vi "statsNsplit2ADC.vi"(4 "Start":i32=200, 5 "Tabin":i32[](array[numeric])=[0, 1, 2, 3, 4, 5, 6, 7, 8, 0, 1, 2, 3, 4, 5, 6, 7, 8], 6 "Nbins":i32=1, 7 "channel nb":u8=8 format="%x") -> (0 "Averages":dbl[][](array[numeric]), 1 "S.Dev.":dbl[][](array[numeric]), 2 "Minima":i32[][](array[numeric]), 3 "Maxima":i32[][](array[numeric]))   [LabVIEW 2014]
uses:
  <vilib>/Analysis/NI_AALBase.lvlib
panel:
  out "subarray":i32[](array[numeric])
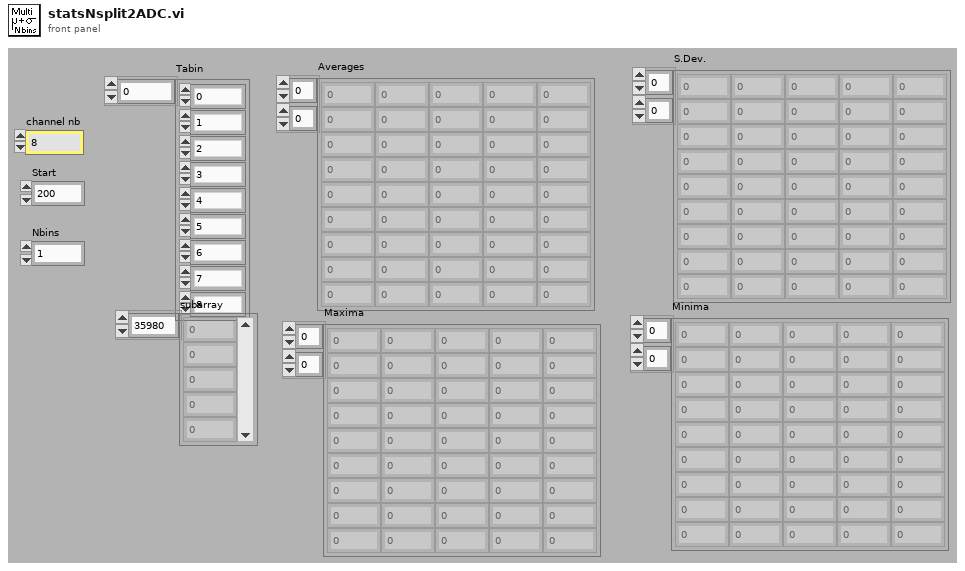
[diagram p1: front panel]
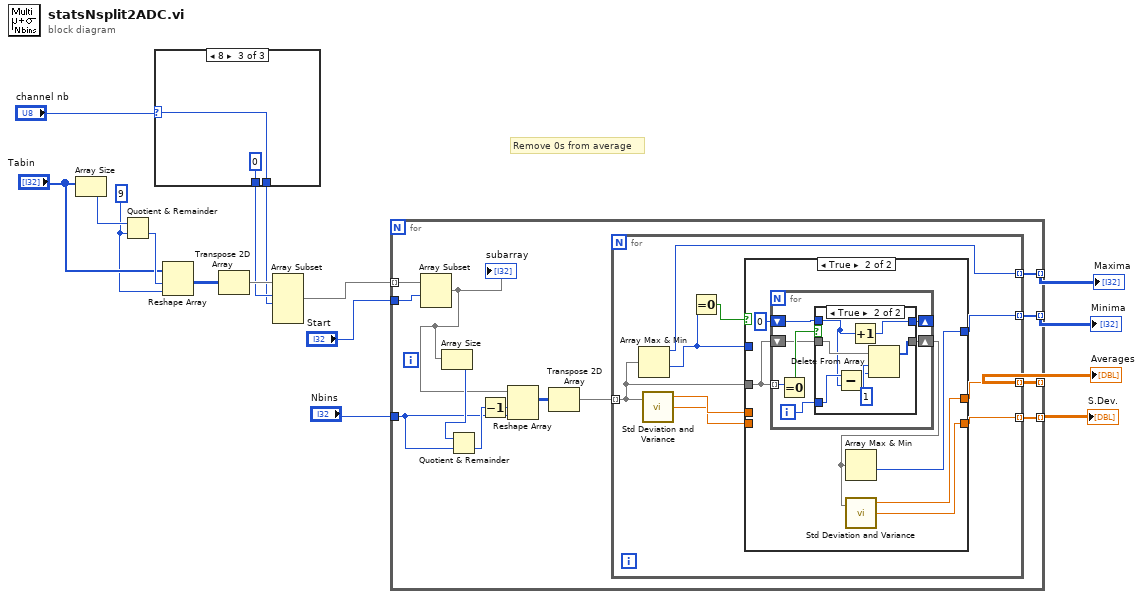
[diagram p0: block diagram]
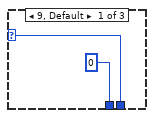
[diagram p2: hidden frame]
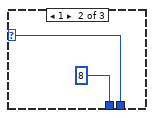
[diagram p3: hidden frame]
diagram:
  w7 = 9
  # "Remove 0s from average"
  n1 = Array Size(array="Tabin") -> (size(s)=w12:i32)
  n2 = Quotient & Remainder(x=w12, y=w7) -> (floor(x/y)=w11:i32)  [unwired: 1 out]
  n3 = case shown="8" "channel nb" {
    selector: "channel nb" -> [w17 w20 w22]
    tunnel: [w17 w20 w22] -> w3
    tunnel: [0 8 0] -> w4
    frame 9, Default {
    }
    frame 1 {
    }
    frame 8 {
    }
  }
  n4 = Reshape Array("Tabin", w11, w7) -> (w9:i32[][])
  n5 = Transpose 2D Array(2D array=w9) -> (transposed array=w8:i32[][])
  n6 = Array Subset(array=w8, index (row)=w4, length (row)=w3) -> (w6:i32[][])  [unwired: 2 in]
  n7 = for {
    tunnel: "Start" -> [w28]
    tunnel: "Nbins" -> [w30]
    tunnel: [w34] -> w14 mode=indexing
    tunnel: [w33] -> w13 mode=indexing
    tunnel: w6 -> [w27] mode=indexing
    tunnel: [w24] -> w2 mode=indexing
    tunnel: [w23] -> w1 mode=indexing
    n8 = Array Subset(array=w27, index=w28) -> (w26:i32[])  [unwired: 1 in]
    "subarray" <- w26
    n9 = Array Size(array=w26) -> (size(s)=w32:i32)
    n10 = Quotient & Remainder(x=w32, y=w30) -> (floor(x/y)=w31:i32)  [unwired: 1 out]
    n11 = Decrement(x=w31) -> (x-1=w25:i32)
    n12 = Reshape Array(w26, w25, w30) -> (w35:i32[][])
    n13 = Transpose 2D Array(2D array=w35) -> (transposed array=w29:i32[][])
    n14 = for {
      tunnel: w29 -> [w36] mode=indexing
      tunnel: [w39] -> w34 mode=indexing
      tunnel: [w37] -> w33 mode=indexing
      tunnel: [w43] -> w24 mode=indexing
      tunnel: [w41] -> w23 mode=indexing
      n15 = Array Max & Min(array=w36) -> (max value=w43:i32, min value=w42:i32)  [unwired: 2 out]
      n16 = call <vilib>:"Std Deviation and Variance.vi"("X"=w36) -> ("mean"=w40:dbl, "standard deviation"=w38:dbl)  [unwired: 1 in, 1 out]
      n17 = Equal To 0?(x=w42) -> (x = 0?=w44:bool)
      n18 = case shown="True" w44 {
        tunnel: w42 -> [w47 _]
        tunnel: [w47 w48] -> w41
        tunnel: w40 -> [w46 _]
        tunnel: [w46 w50] -> w39
        tunnel: w38 -> [w45 _]
        tunnel: [w45 w49] -> w37
        tunnel: w36 -> [_ w53]
        frame False {
        }
        frame True {
          n19 = for {
            tunnel: w53 -> [w60] mode=indexing
            shift-right: [w54] -> w51
            shift-left: w53 -> [w56]
            shift-right: [w57] -> _
            shift-left: 0 -> [w58]
            i -> [w55]
            n20 = Equal To 0?(x=w60) -> (x = 0?=w59:bool)
            n21 = case shown="True" w59 {
              tunnel: w58 -> [w62 w65]
              tunnel: [w62 w69] -> w57
              tunnel: w56 -> [w61 w68]
              tunnel: w55 -> [_ w66]
              tunnel: [w61 w63] -> w54
              frame False {
              }
              frame True {
                n22 = Subtract(x=w66, y=w65) -> (x-y=w64:i32)
                n23 = Increment(x=w65) -> (x+1=w69:i32)
                n24 = Delete From Array(array=w68, length=1, index=w64) -> (array with subset deleted=w63:i32[])  [unwired: 1 out]
              }
            }
          }
          n25 = Array Max & Min(array=w51) -> (min value=w48:i32)  [unwired: 3 out]
          n26 = call <vilib>:"Std Deviation and Variance.vi"("X"=w51) -> ("mean"=w50:dbl, "standard deviation"=w49:dbl)  [unwired: 1 in, 1 out]
        }
      }
    }
  }
  "Averages" <- w14
  "S.Dev." <- w13
  "Maxima" <- w2
  "Minima" <- w1
